vi "Autobuild Main.vi"() -> ()   [LabVIEW 2022 SP3]
uses:
  subVIs/Package Builder API/build type.ctl
  subVIs/Package Builder API/NI Package Builder API.lvlib
panel:
  in  "Build Package":bool=TRUE
  in  "Build EXEs":bool=TRUE
  out "Current Build":i32
  out "Total to Build":i32
  in  "Tab Control":T1(tab)
  in  "Projects":path[](array[path])=[path "C:/dev/digital-microphone/source/frequency response/Frequency Response.lvproj", path "C:/dev/digital-microphone/source/single tone/Single Tone.lvproj", path "C:/dev/digital-microphone/source/calibrate acoustic output/Calibrate Acoustic Output.lvproj"]
  out "command line standard output":string
  in  "package builder solution path":path=path "C:/dev/digital-microphone/package/DigitalMicrophone.pbs"
  in  "error in (no error)":errorcluster
  out "error out":errorcluster
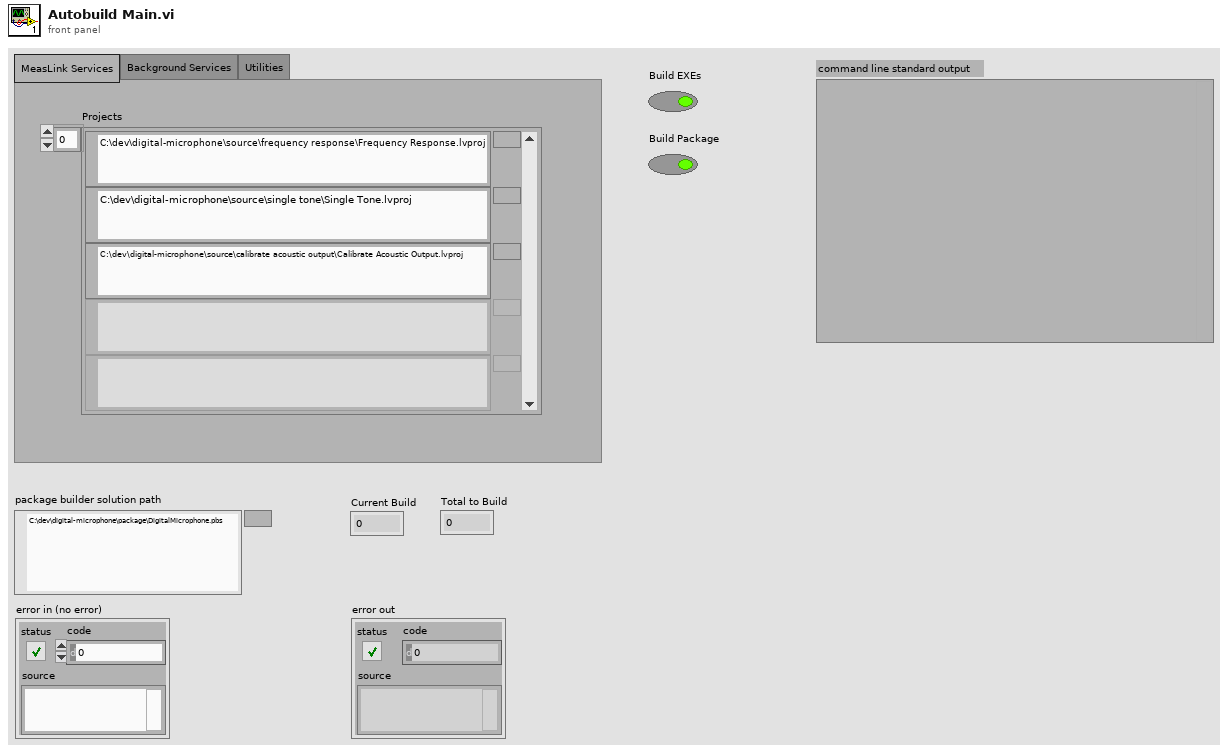
[diagram p1: front panel]
types:
  T1 = enum32{"MeasLink Services", "Background Services", "Utilities"}
  T2 = typedef "NI Package Builder API.lvlib/build type.ctl" = enum16{"packages", "feeds", "solution"}
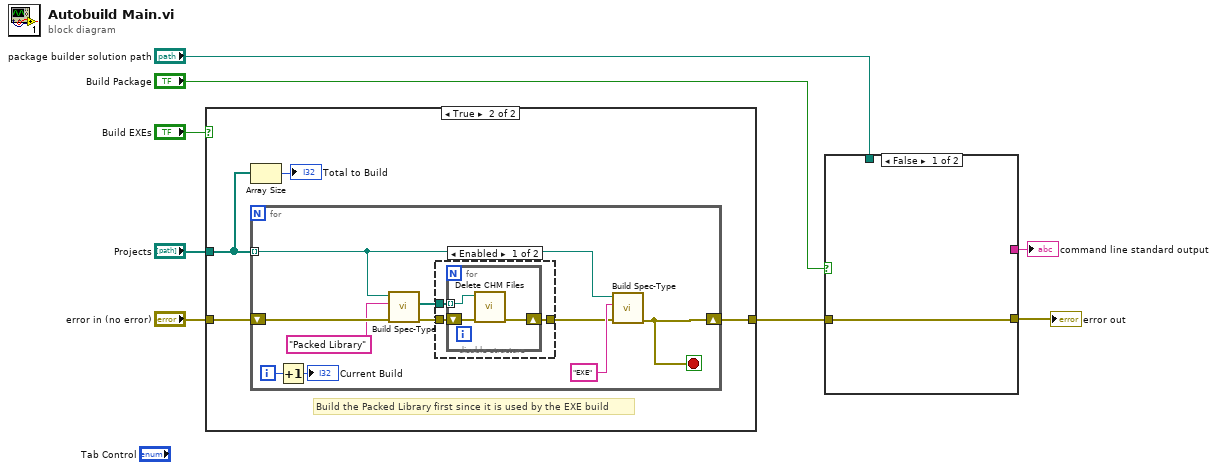
[diagram p0: block diagram]
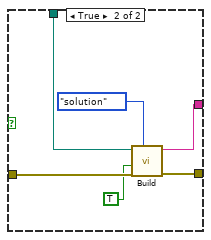
[diagram p4: hidden frame]
diagram:
  n1 = case shown="True" "Build EXEs" {
    tunnel: "error in (no error)" -> [w9 w13]
    tunnel: [w9 w12] -> w4
    tunnel: "Projects" -> [_ w11]
    frame False {
    }
    frame True {
      # "Build the Packed Library first since it is used by the EXE build"
      n2 = Array Size(array=w11) -> (size(s)=→"Total to Build":i32)
      n3 = for {
        shift-right: [w16] -> w12
        shift-left: w13 -> [w23]
        tunnel: w11 -> [w20] mode=indexing
        i -> [w15]
        stop <- w16 stop-if-true
        n4 = Increment(x=w15) -> (x+1=→"Current Build":i32)
        n5 = call "Build Spec-Type.vi"("error in (no error)"=w23, "Type"="Packed Library", "Path to project"=w20) -> ("error out"=w19:errorcluster, "Generated files"=w17:path[])  [unwired: 7 in]
        n6 = disable-structure shown="Enabled" {
          disable-tunnel: w19 -> [w26 w30]
          disable-tunnel: [w25 w30] -> w18
          disable-tunnel: w17 -> [w24 _]
          frame Enabled {
            n7 = for {
              shift-right: [w28] -> w25
              shift-left: w26 -> [w29]
              tunnel: w24 -> [w27] mode=indexing
              n8 = call "Delete CHM Files.vi"("error in (no error)"=w29, "Path"=w27) -> ("error out"=w28:errorcluster)  [unwired: 9 in]
            }
          }
          frame Disabled {
          }
        }
        n9 = call "Build Spec-Type.vi"("error in (no error)"=w18, "Type"="EXE", "Path to project"=w20) -> ("error out"=w16:errorcluster)  [unwired: 7 in, 1 out]
      }
    }
  }
  n10 = case shown="False" "Build Package" {
    tunnel: [w31 w37] -> w8
    tunnel: "package builder solution path" -> [_ w36]
    tunnel: [_ w35] -> w6
    tunnel: w4 -> [w31 w34]
    frame False {
    }
    frame True {
      n11 = call "Build.vi"("bulid type"=build_type."solution", "error in (no error)"=w34, "save build info to solution"=TRUE, "package builder solution path"=w36) -> ("error out"=w37:errorcluster, "command line standard output"=w35:string)  [unwired: 6 in]
    }
  }
  "error out" <- w8
  "command line standard output" <- w6
